vi "GetClampResultValue.vi"(8 "error in (no error)":errorcluster, 9 "data":T1={"Points"=[], "Perpendicular Lines"=[], "appended array"=[], "Line Coordinates"=[], "Clamp Settings"={"Contrast"=0, "Filter width"=0, "Steepness"=0, "Subsampling Ratio"=0, "Show Search Area"=FALSE, "Show Search Lines"=FALSE, "Show Edges Found"=FALSE, "Show Result"=FALSE}, "ROI Descriptor"={"Global Rectangle"=[], "Contours"=[]}, "Distance"=0.0, "Edge Coordinates"=[{"X"=441.67966, "Y"=663.0}, {"X"=684.4586, "Y"=655.0}], "Edge Coordinates  (Real World)"=[{"X"=441.67966, "Y"=663.0}, {"X"=684.4586, "Y"=655.0}], "Distance (Real World)"=0.0}, 11 "Analysis_Clamp_Parameter":T2={"Clamp Settings"={"Contrast"=40, "Filter width"=4, "Steepness"=2, "Subsampling Ratio"=5, "Show Search Area"=TRUE, "Show Search Lines"=TRUE, "Show Edges Found"=TRUE, "Show Result"=TRUE}, "ROI Descriptor"={"Global Rectangle"=[], "Contours"=[]}, "Process"=0}) -> (0 "error out":errorcluster, 3 "ResultValues":string[](array[string]))   [LabVIEW 2019]
uses:
  Controls/Clamp/Analysis_Clamp_Parameter.ctl
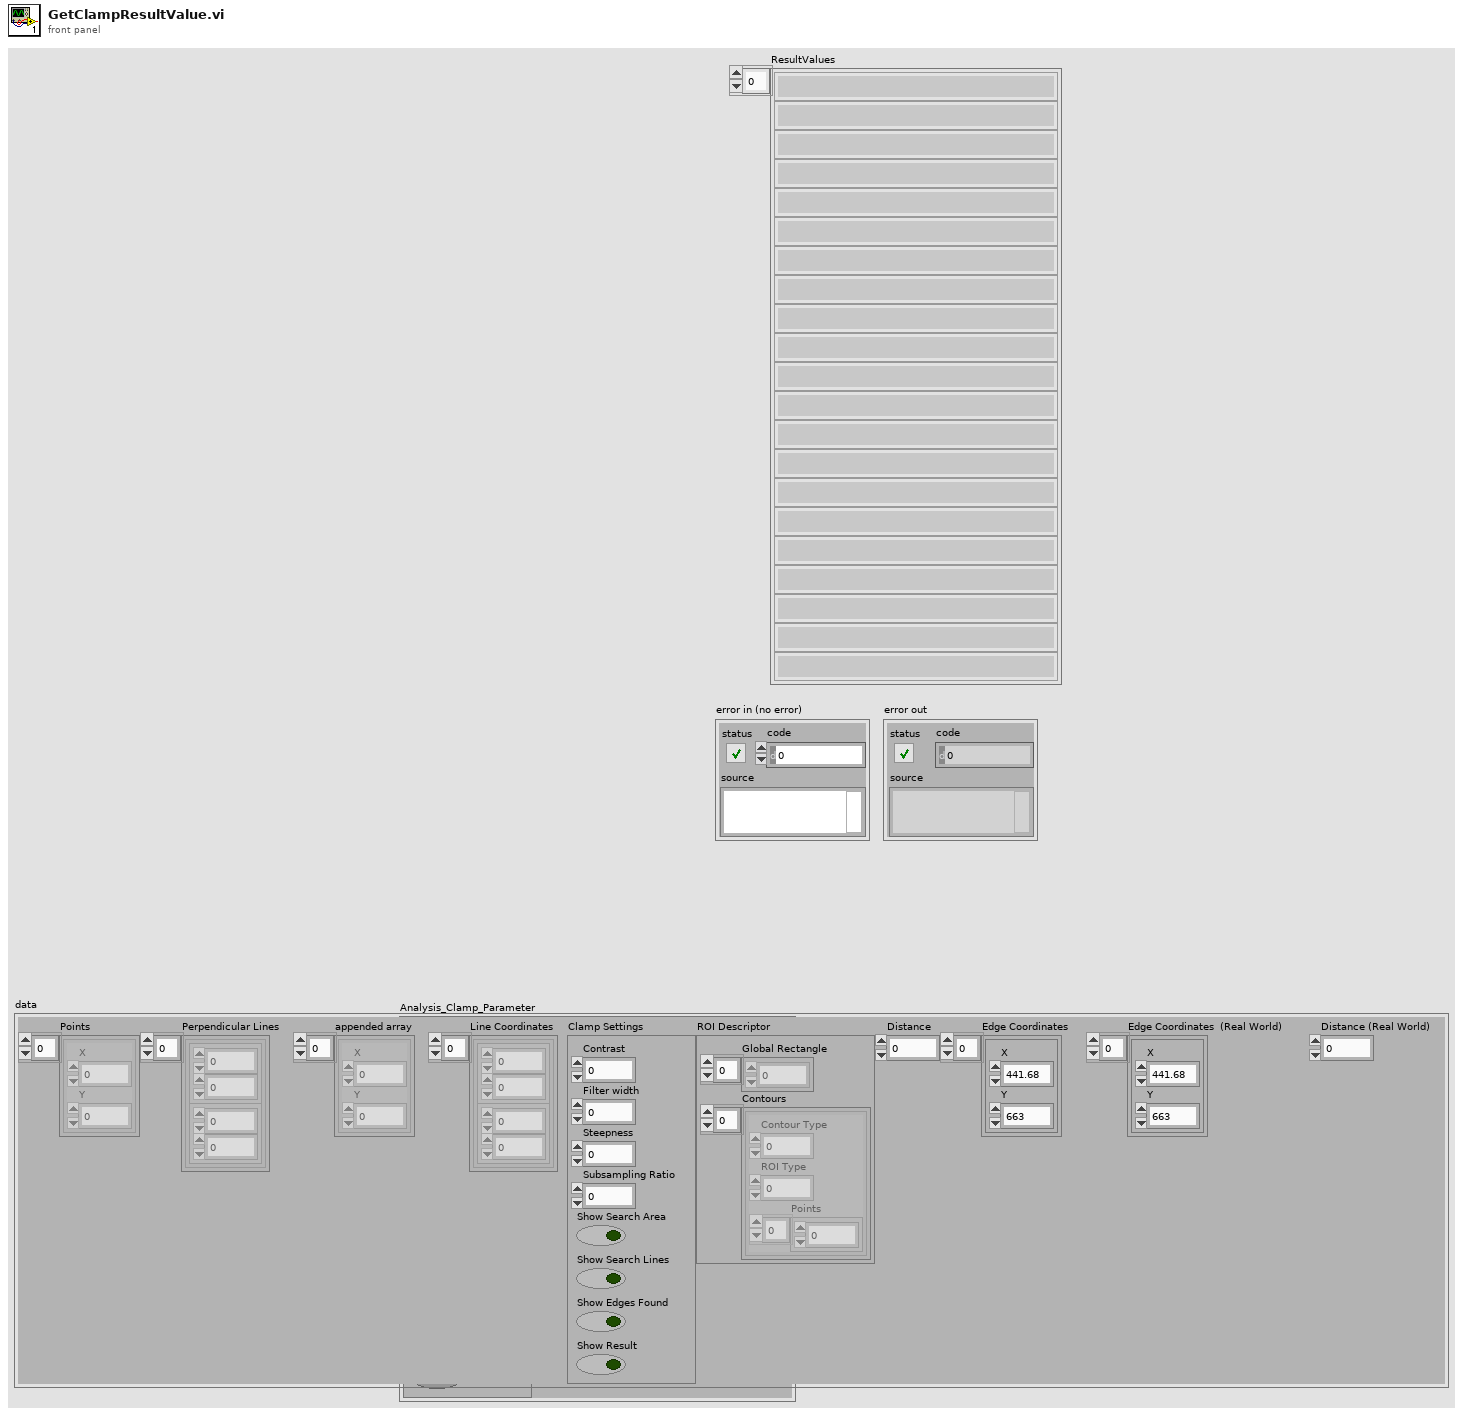
[diagram p1: front panel]
types:
  T1 = cluster{"Points":cluster{"X":sgl, "Y":sgl}[], "Perpendicular Lines":cluster{cluster{sgl, sgl}, cluster{sgl, sgl}}[], "appended array":cluster{"X":sgl, "Y":sgl}[], "Line Coordinates":cluster{cluster{sgl, sgl}, cluster{sgl, sgl}}[], "Clamp Settings":cluster{"Contrast":i32, "Filter width":i32, "Steepness":i32, "Subsampling Ratio":u32, "Show Search Area":bool, "Show Search Lines":bool, "Show Edges Found":bool, "Show Result":bool}, "ROI Descriptor":cluster{"Global Rectangle":i32[], "Contours":cluster{"Contour Type":u32, "ROI Type":u32, "Points":i32[]}[]}, "Distance":sgl, "Edge Coordinates":cluster{"X":sgl, "Y":sgl}[], "Edge Coordinates  (Real World)":cluster{"X":sgl, "Y":sgl}[], "Distance (Real World)":sgl}
  T2 = typedef "Analysis_Clamp_Parameter.ctl" = cluster{"Clamp Settings":cluster{"Contrast":i32, "Filter width":i32, "Steepness":i32, "Subsampling Ratio":u32, "Show Search Area":bool, "Show Search Lines":bool, "Show Edges Found":bool, "Show Result":bool}, "ROI Descriptor":cluster{"Global Rectangle":i32[], "Contours":cluster{"Contour Type":u32, "ROI Type":u32, "Points":i32[]}[]}, "Process":u16}
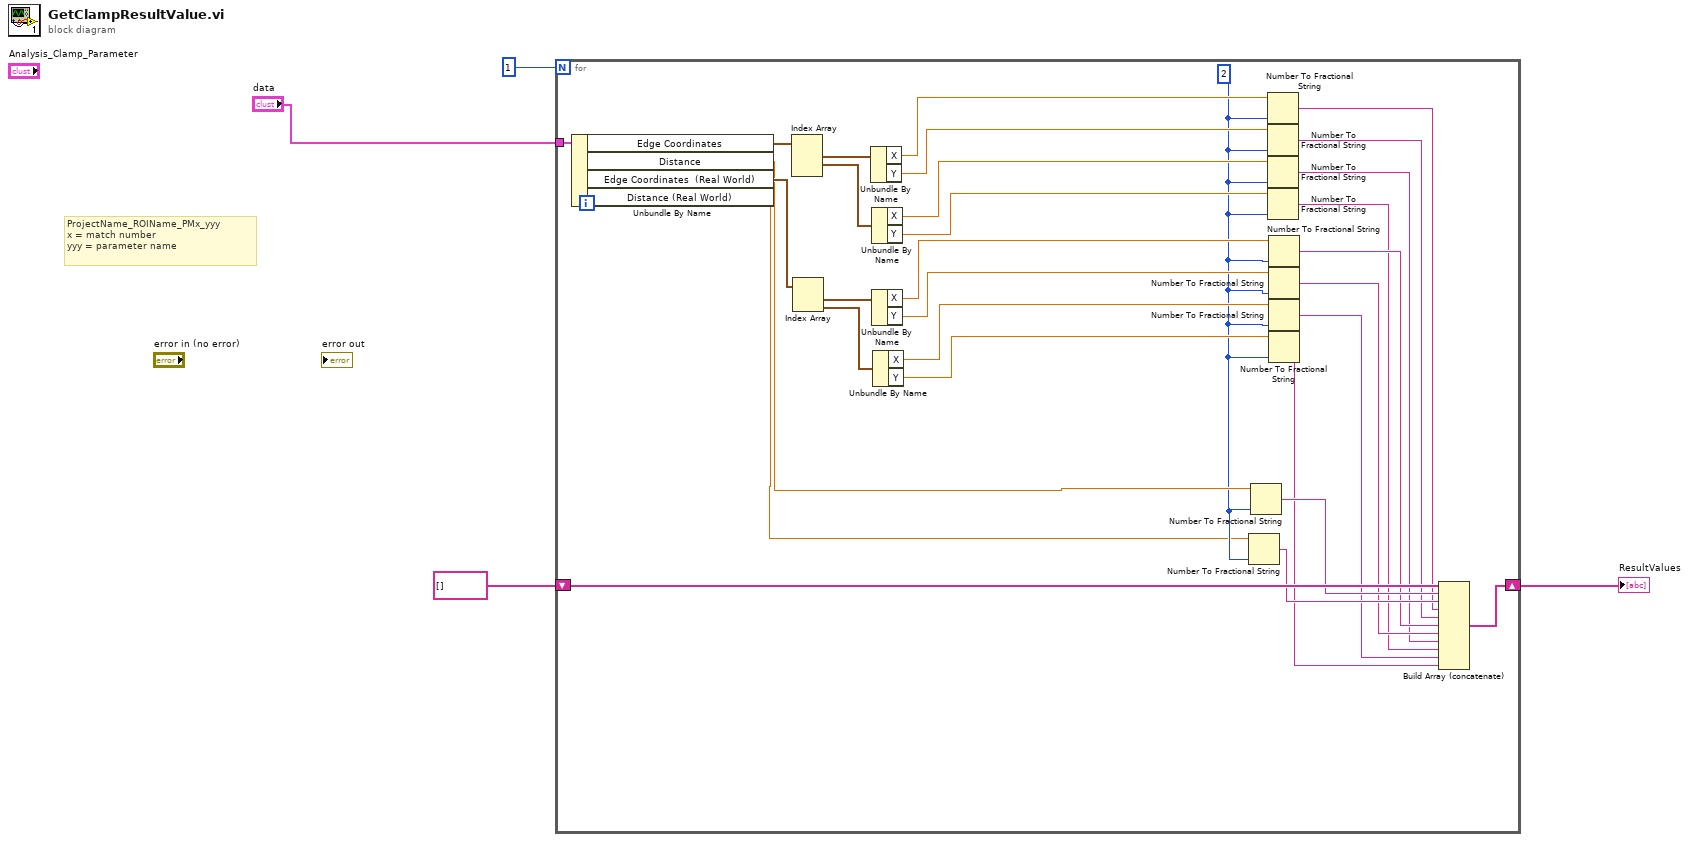
[diagram p0: block diagram]
diagram:
  # "ProjectName_ROIName_PMx_yyy\nx = match number\nyyy = parameter name"
  n1 = for {
    N: 1 ("Number of Matches Requested") -> [_]
    shift-right: [w32] -> w3
    shift-left: string[] [] -> [w33]
    tunnel: "data" -> [w34]
    w15 = 2
    n2 = Unbundle By Name(w34) -> ("Edge Coordinates"=w31:cluster{"X":sgl, "Y":sgl}[], "Distance"=w16:sgl, "Edge Coordinates  (Real World)"=w17:cluster{"X":sgl, "Y":sgl}[], "Distance (Real World)"=w14:sgl)
    n3 = Index Array(array=w31) -> (element #1=w30:cluster{"X":sgl, "Y":sgl}, element #2=w29:cluster{"X":sgl, "Y":sgl})  [unwired: 3 in, 1 out]
    n4 = Index Array(array=w17) -> (element #1=w18:cluster{"X":sgl, "Y":sgl}, element #2=w19:cluster{"X":sgl, "Y":sgl})  [unwired: 2 in]
    n5 = Unbundle By Name(w30) -> ("X"=w28:sgl, "Y"=w27:sgl)
    n6 = Unbundle By Name(w29) -> ("X"=w26:sgl, "Y"=w25:sgl)
    n7 = Unbundle By Name(w18) -> ("X"=w20:sgl, "Y"=w21:sgl)
    n8 = Unbundle By Name(w19) -> ("X"=w22:sgl, "Y"=w23:sgl)
    n9 = Number To Fractional String(number=w14, precision (6)=w15) -> (F-format string=w13:string)  [unwired: 2 in]
    n10 = Number To Fractional String(number=w16, precision (6)=w15) -> (F-format string=w24:string)  [unwired: 2 in]
    n11 = Number To Fractional String(number=w28, precision (6)=w15) -> (F-format string=w12:string)  [unwired: 2 in]
    n12 = Number To Fractional String(number=w27, precision (6)=w15) -> (F-format string=w11:string)  [unwired: 2 in]
    n13 = Number To Fractional String(number=w26, precision (6)=w15) -> (F-format string=w8:string)  [unwired: 2 in]
    n14 = Number To Fractional String(number=w25, precision (6)=w15) -> (F-format string=w7:string)  [unwired: 2 in]
    n15 = Number To Fractional String(number=w20, precision (6)=w15) -> (F-format string=w10:string)  [unwired: 2 in]
    n16 = Number To Fractional String(number=w21, precision (6)=w15) -> (F-format string=w9:string)  [unwired: 2 in]
    n17 = Number To Fractional String(number=w22, precision (6)=w15) -> (F-format string=w6:string)  [unwired: 2 in]
    n18 = Number To Fractional String(number=w23, precision (6)=w15) -> (F-format string=w5:string)  [unwired: 2 in]
    n19 = Build Array (concatenate)(w33, w24, w13, w12, w11, w10, w9, w8, w7, w6, w5) -> (w32:string[])
  }
  "ResultValues" <- w3
